vi "CAN TPCANHandle-Bitrate-from-Enum.vi"(11 "TPCANHandle-Bitrate":T1) -> (3 "Btr0Btr1":u16)   [LabVIEW 2020, in "PCANBasic_eX.lvlib"]
uses:
  PCANBasic_eX.lvlib
  CTLs/TPCANHandle-Bitrate_eX.ctl
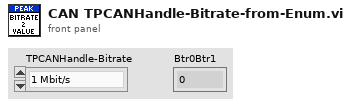
[diagram p1: front panel]
types:
  T1 = typedef "PCANBasic_eX.lvlib/TPCANHandle-Bitrate_eX.ctl" = enum16{"1 Mbit/s", "800 KBit/s", "500 KBit/s", "250 KBit/s", "125 KBit/s", "100 KBit/s"}
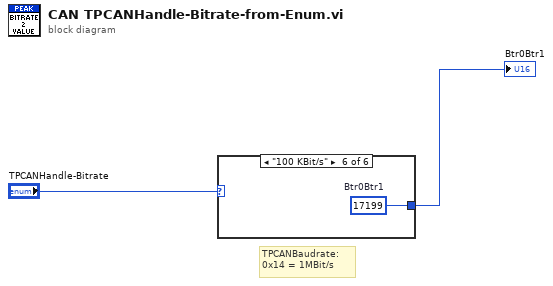
[diagram p0: block diagram]
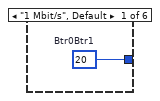
[diagram p2: hidden frame]
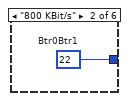
[diagram p3: hidden frame]
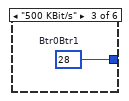
[diagram p4: hidden frame]
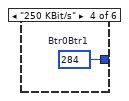
[diagram p5: hidden frame]
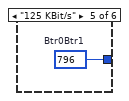
[diagram p6: hidden frame]
diagram:
  # "TPCANBaudrate:\n0x14 = 1MBit/s"
  n1 = case shown="\"100 KBit/s\"" "TPCANHandle-Bitrate" {
    tunnel: [w3 w4 w5 w6 w7 w8] -> w1
    frame "1 Mbit/s", Default {
      w3 = u16 20  # Btr0Btr1
    }
    frame "800 KBit/s" {
      w4 = u16 22  # Btr0Btr1
    }
    frame "500 KBit/s" {
      w5 = u16 28  # Btr0Btr1
    }
    frame "250 KBit/s" {
      w6 = u16 284  # Btr0Btr1
    }
    frame "125 KBit/s" {
      w7 = u16 796  # Btr0Btr1
    }
    frame "100 KBit/s" {
      w8 = u16 17199  # Btr0Btr1
    }
  }
  "Btr0Btr1" <- w1
